vi "Pre-start common checks logic.vi"() -> (3 "Proceed":bool)   [LabVIEW 2013]
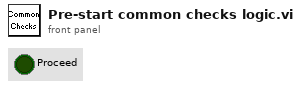
[diagram p1: front panel]
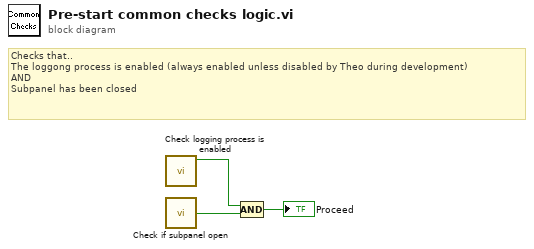
[diagram p0: block diagram]
diagram:
  # "Checks that..\nThe loggong process is enabled (always enabled unless disabled by Theo during development)\nAND\nSubpanel has been closed"
  n1 = call "Check logging process is enabled.vi"() -> ("Proceed / Logging process is enabled"=w1:bool)  [unwired: 11 in]
  n2 = call "Check if subpanel open.vi"() -> ("Proceed / Subpanel is not open"=w2:bool)  [unwired: 1 in]
  n3 = Compound Arithmetic op=AND(w1, w2) -> (→"Proceed":bool)
